vi "Create Instrument Addon From Configuration File_ex.vi"() -> ()   [LabVIEW 2019]
uses:
  NationalInstruments.VeriStand.SystemDefinitionAPI
  <vilib>/NI VeriStand/Custom Device API/Custom Device Item Ref.ctl
  Control 2.ctl
  Addon/Support Libraries/Protocols.lvlibp/Protocol Parent/Protocol Parent.lvclass
  Scripting API/Scripting API.lvlib
  <vilib>/NI VeriStand/Custom Device API/Custom Device API.lvlib
panel:
  out "Target Out":refnum<k24>
  out "Instrument Addon Refnum":T1=18446744073709551615 format="%.0x"
  out "Message Channels Refnums":T2 {"Enable Periodic" format="%.0x"; "Error Code" format="%.0x"; "Message Status" format="%.0x"; "Timestamp" format="%.0x"; "Trigger" format="%.0x"}
  out "Error Out":errorcluster
  in  "Config File Path":path
  in  "Error In":errorcluster
  in  "Target In":refnum<k24>
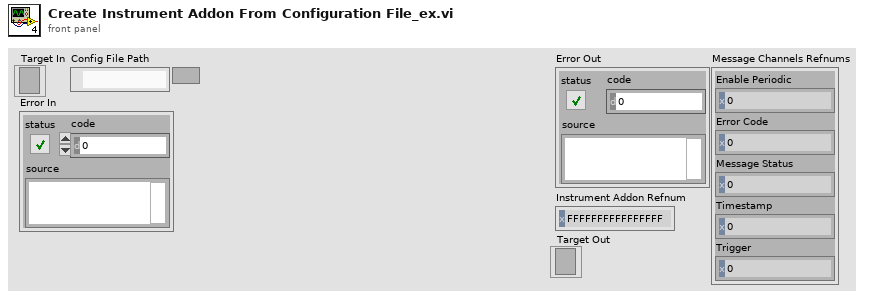
[diagram p1: front panel]
types:
  T1 = typedef "Custom Device API.lvlib/Custom Device Item Ref.ctl" = u64
  T2 = cluster{"Enable Periodic":T1, "Error Code":T1, "Message Status":T1, "Timestamp":T1, "Trigger":T1}
  T3 = typedef "Control 2.ctl" = cluster{"Protocol":refnum<class "Protocol Parent.lvclass">, "PCL Decimation":u16}
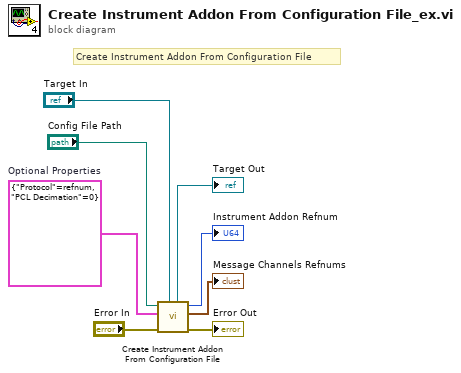
[diagram p0: block diagram]
diagram:
  w1 = T3 {"Protocol"=refnum, "PCL Decimation"=0}  # Optional Properties
  # "Create Instrument Addon From Configuration File"
  n1 = call "Create Instrument Addon From Configuration File.vi"("Target In"="Target In", "Error In"="Error In", "Optional Properties"=w1, "Config File Path"="Config File Path") -> ("Error Out"=→"Error Out":errorcluster, "Message Channels refnums"=→"Message Channels Refnums":T2, "Instrument Addon Refnum"=→"Instrument Addon Refnum":T1, "Target Out"=→"Target Out":refnum<k24>)  [unwired: 4 in]
